vi "RT Driver VI.vi"(7 "Operation":T1, 11 "Device Reference in":T2 format="%.0x") -> (0 "Error Code":i32)   [LabVIEW 2017, in "NI-XNET Monitor Engine.lvlib"]
uses:
  NI-XNET Monitor Engine.lvlib
  <vilib>/NI Veristand/Custom Device API/Custom Device Item Ref.ctl
  <vilib>/NI Veristand/Custom Device API/Hardware Interface Driver VI Operation.ctl
  RTStateVariables.ctl
  <vilib>/NI/NIVS Inline Async API/_VS Inline Async API/VS Inline Async API/VS Inline Async API.lvclass
  Shared/Compiled.Data.ctl
  <vilib>/NI/NIVS Inline Async API/_VS Inline Async API/VS Inline Async API/VS Inline Async API.lvclass/VS Inline Async API.ctl
  <vilib>/NI/NIVS Inline Async API/_Data Access Engine/Data Access Engine/Data Access Engine.lvclass/Data Access Engine.ctl
  <vilib>/NI/NIVS Inline Async API/_Data Access Engine/Access Type Classes/Write/Write.lvclass/Write.ctl
  <vilib>/NI/NIVS Inline Async API/_Data Access Engine/Access Type Classes/ReadWrite/ReadWrite.lvclass/ReadWrite.ctl
  <vilib>/NI/NIVS Inline Async API/_Data Access Engine/Data Access Engine/Methods/Data.Engine.Read Data from HW.vi
  <vilib>/NI/NIVS Inline Async API/_VS Inline Async API/Error Handling Process/SubVIs/Error.GetError.vi
  <vilib>/NI/NIVS Inline Async API/_Data Access Engine/Access Type Classes/ReadWrite/ReadWrite.EngineData.vi
  <vilib>/NI/NIVS Inline Async API/_Data Access Engine/Access Type Classes/Write/Write.EngineData.vi
  <vilib>/NI Veristand/Custom Device API/NI VeriStand - Get Channel Value by Data Reference.vi
  <vilib>/NI Veristand/Custom Device API/NI VeriStand - Set Channel Value by Data Reference.vi
  Shared/Constants.vi
  <vilib>/NI Veristand/Custom Device API/Get Item Property (Variant).vi
  <vilib>/NI Veristand/Custom Device API/Global Data Refs.vi
  <vilib>/NI Veristand/Custom Device API/Custom Device API.lvlib
  <vilib>/NI VeriStand/Custom Device Tools/Custom Device Utility Library/Custom Device Utility Library.lvlib
  Shared/NI-XNET Monitor Shared.lvlib
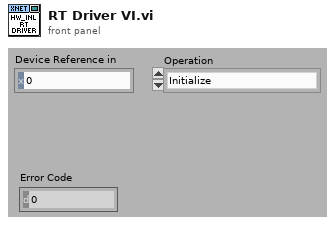
[diagram p1: front panel]
types:
  T1 = typedef "Custom Device API.lvlib/Hardware Interface Driver VI Operation.ctl" = enum16{"Initialize", "Start", "Read Data from HW", "Write Data to HW", "Close"}
  T2 = typedef "Custom Device API.lvlib/Custom Device Item Ref.ctl" = u64
  T3 = typedef "NI-XNET Monitor Engine.lvlib/RTStateVariables.ctl" = cluster{"Async":refnum<class "VS Inline Async API.lvclass">, "Settings":T4}
  T4 = typedef "NI-XNET Monitor Shared.lvlib/Compiled.Data.ctl" = cluster{"CAN":string[], "FlexRay":string[], "LIN":string[], "Async Loop Rate (s)":dbl}
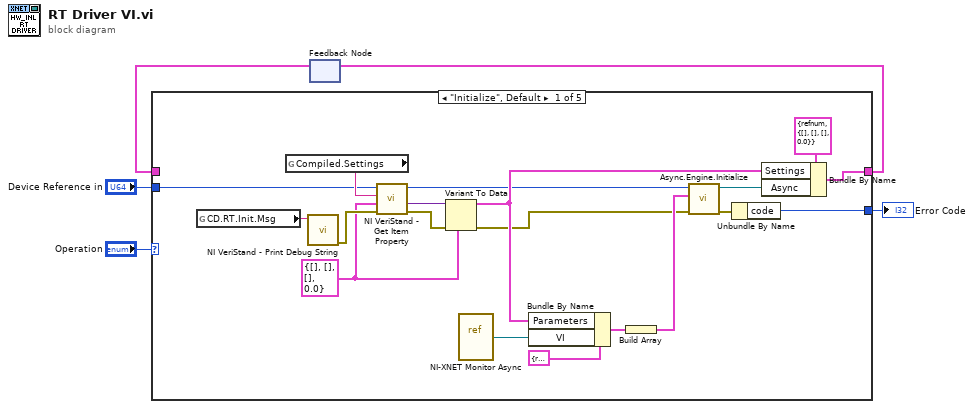
[diagram p0: block diagram]
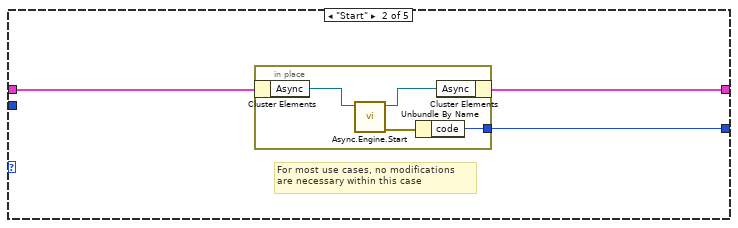
[diagram p2: hidden frame]
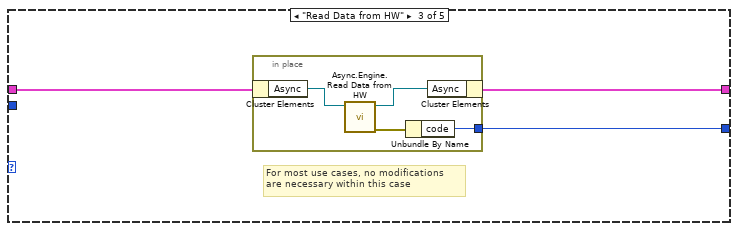
[diagram p3: hidden frame]
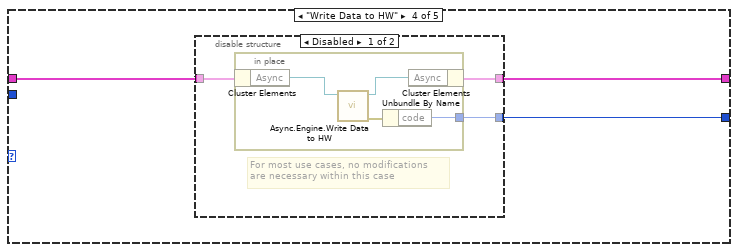
[diagram p4: hidden frame]
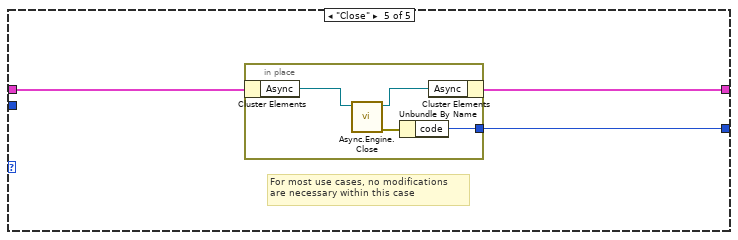
[diagram p6: hidden frame]
diagram:
  n1 = feedback #1() -> (w3:T3)  [unwired: 1 out]
  n2 = case shown="\"Initialize\", Default" "Operation" {
    tunnel: [w22 w26 w32 w39 w51] -> w4
    tunnel: w3 -> [_ w27 w34 w40 w52]
    tunnel: "Device Reference in" -> [w6 _ _ _ _]
    tunnel: [w24 w25 w33 w41 w50] -> w1
    frame "Initialize", Default {
      w11 = T4 {"CAN"=[], "FlexRay"=[], "LIN"=[], "Async Loop Rate (s)"=0.0} ("Settings")
      n3 = global read "Constants.vi" "CD.RT.Init.Msg"() -> (w7:string)
      n4 = global read "Constants.vi" "Compiled.Settings"() -> (w10:string)
      n5 = call <vilib>:"NI VeriStand - Print Debug String.vi"("Message"=w7) -> ("error out"=w14:errorcluster)  [unwired: 10 in]
      n6 = call-poly <vilib>:"NI VeriStand - Get Item Property.vi"("error in (no error)"=w14, "Default Value"=w11, "Property Name"=w10, "Item Ref in"=w6) -> ("error out"=w19:errorcluster, "Value"=w18:variant, "Item Ref out"=w15:T2)  [unwired: 4 in, 1 out]
      n7 = Variant To Data(error in=w19, type=w11, Variant=w18) -> (data=w16:T4, error out=w9:errorcluster)
      n8 = vi-ref "NI-XNET Monitor Async.vi"() -> (w13:refnum<vi>)
      n9 = Bundle By Name(cluster=cluster{"VI":refnum<vi>, "Parameters":variant} {"VI"=refnum, "Parameters"=variant} ("Process"), "Parameters"=w16, "VI"=w13) -> (w20:cluster{"VI":refnum<vi>, "Parameters":variant})
      n10 = Build Array(w20) -> (w17:cluster{"VI":refnum<vi>, "Parameters":variant}[])
      n11 = call <vilib>:"Async.Engine.Initialize.vi"("error in (no error)"=w9, "Processes"=w17, "Custom Device Ref"=w15) -> ("error out"=w8:errorcluster, "Async"=w23:refnum<class "VS Inline Async API.lvclass">)  [unwired: 7 in]
      n12 = Unbundle By Name(w8) -> ("code"=w24:i32)
      n13 = Bundle By Name(cluster=T3 {"Async"=refnum, "Settings"={"CAN"=[], "FlexRay"=[], "LIN"=[], "Async Loop Rate (s)"=0.0}} ("RT State Variables"), "Settings"=w16, "Async"=w23) -> (w22:T3)
    }
    frame "Start" {
      # "For most use cases, no modifications \nare necessary within this case"
      n14 = in-place {
        in-place-border: [w28] -> w25
        n15 = in-place-cluster #2(w27) -> ("Async"=w31:refnum<class "VS Inline Async API.lvclass">)
        n16 = call <vilib>:"Async.Engine.Start.vi"("VS Inline Async API in"=w31) -> ("error out"=w29:errorcluster, "VS Inline Async API out"=w30:refnum<class "VS Inline Async API.lvclass">)  [unwired: 9 in]
        n17 = Unbundle By Name(w29) -> ("code"=w28:i32)
        n18 = in-place-cluster #2("Async"=w30) -> (w26:T3)
      }
    }
    frame "Read Data from HW" {
      # "For most use cases, no modifications \nare necessary within this case"
      n19 = in-place {
        in-place-border: [w38] -> w33
        n20 = in-place-cluster #3(w34) -> ("Async"=w37:refnum<class "VS Inline Async API.lvclass">)
        n21 = call <vilib>:"Async.Engine.Read Data from HW.vi"("Async in"=w37) -> ("error out"=w35:errorcluster, "Async out"=w36:refnum<class "VS Inline Async API.lvclass">)  [unwired: 9 in]
        n22 = Unbundle By Name(w35) -> ("code"=w38:i32)
        n23 = in-place-cluster #3("Async"=w36) -> (w32:T3)
      }
    }
    frame "Write Data to HW" {
      n24 = disable-structure shown="Disabled" {
        disable-tunnel: [w44 _] -> w41
        disable-tunnel: w40 -> [w43 w49]
        disable-tunnel: [w42 w49] -> w39
        frame Disabled {
          # "For most use cases, no modifications \nare necessary within this case"
          n25 = in-place {
            in-place-border: [w48] -> w44
            n26 = in-place-cluster #4(w43) -> ("Async"=w46:refnum<class "VS Inline Async API.lvclass">)
            n27 = call <vilib>:"Async.Engine.Write Data to HW.vi"("VS Inline Async API in"=w46) -> ("error out"=w47:errorcluster, "VS Inline Async API out"=w45:refnum<class "VS Inline Async API.lvclass">)  [unwired: 9 in]
            n28 = Unbundle By Name(w47) -> ("code"=w48:i32)
            n29 = in-place-cluster #4("Async"=w45) -> (w42:T3)
          }
        }
        frame Enabled {
        }
      }
    }
    frame "Close" {
      # "For most use cases, no modifications \nare necessary within this case"
      n30 = in-place {
        in-place-border: [w54] -> w50
        n31 = in-place-cluster #5(w52) -> ("Async"=w56:refnum<class "VS Inline Async API.lvclass">)
        n32 = call <vilib>:"Async.Engine.Close.vi"("Async in"=w56) -> ("error out"=w53:errorcluster, "Async out"=w55:refnum<class "VS Inline Async API.lvclass">)  [unwired: 9 in]
        n33 = Unbundle By Name(w53) -> ("code"=w54:i32)
        n34 = in-place-cluster #5("Async"=w55) -> (w51:T3)
      }
    }
  }
  "Error Code" <- w1
  n35 = feedback-in #1(w4) -> ()
